vi "gnome sort.vi"(1 "Array in":dbl[](array[numeric])) -> (0 "Array out":dbl[](array[numeric]))   [LabVIEW 2009]
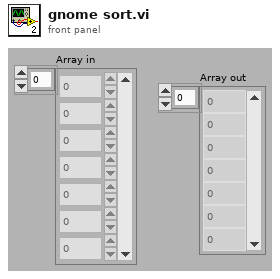
[diagram p1: front panel]
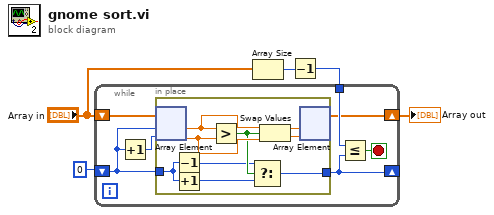
[diagram p0: block diagram]
diagram:
  n1 = Array Size(array="Array in") -> (size(s)=w4:i32)
  n2 = Decrement(x=w4) -> (x-1=w1:i32)
  n3 = while {
    shift-right: [w8] -> _
    shift-left: 0 -> [w10]
    shift-right: [w6] -> w2
    shift-left: "Array in" -> [w12]
    tunnel: w1 -> [w7]
    stop <- w9 stop-if-true
    n4 = Increment(x=w10) -> (x+1=w11:i32)
    n5 = in-place {
      in-place-border: w10 -> [w16]
      in-place-border: [w13] -> w8
      n6 = in-place-array #1(w12, w10, w11) -> (w20:dbl, w21:dbl)
      n7 = Decrement(x=w16) -> (x-1=w14:i32)
      n8 = Increment(x=w16) -> (x+1=w15:i32)
      n9 = Greater?(x=w20, y=w21) -> (0:w19:bool)
      n10 = Select(t=w14, s=w19, f=w15) -> (s? t:f=w13:i32)
      n11 = Swap Values(12:w20, 13:w19, 14:w21) -> (1:w18:dbl, 3:w17:dbl)
      n12 = in-place-array #1(w18, w17) -> (w6:dbl[])  [unwired: 2 out]
    }
    n13 = Less Or Equal?(x=w7, y=w8) -> (x <= y?=w9:bool)
  }
  "Array out" <- w2
